vi "Launcher Views.vi"(8 "error in (no error)":errorcluster, 11 "Abstruct View in":refnum<class "Abstruct View.lvclass">) -> (0 "error out":errorcluster, 3 "Abstruct View out":refnum<class "Abstruct View.lvclass">)   [LabVIEW 2020]
uses:
  Abstruct View.lvclass
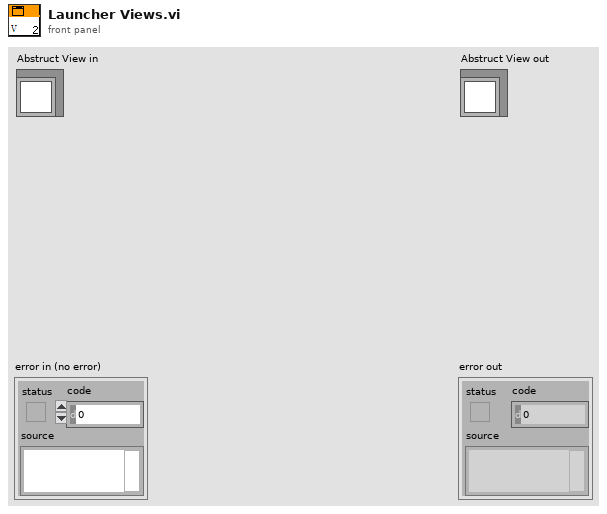
[diagram p1: front panel]
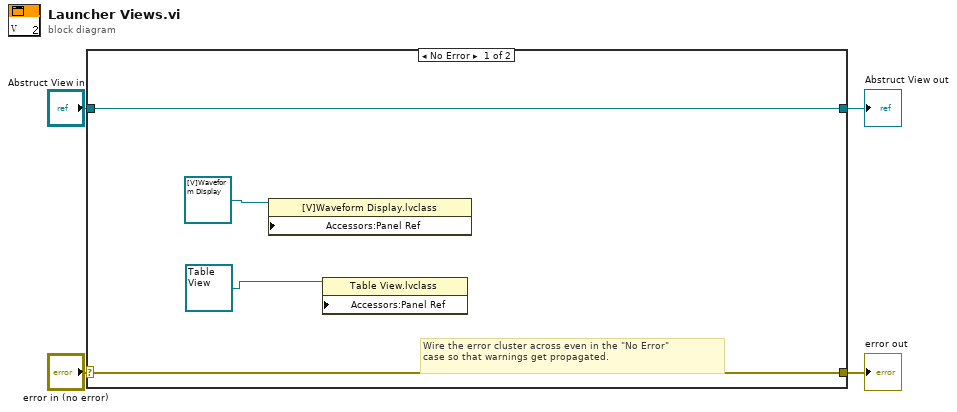
[diagram p0: block diagram]
diagram:
  n1 = case shown="No Error" "error in (no error)" {
    selector: "error in (no error)" -> [w7 w10]
    tunnel: [w7 w10] -> w3
    tunnel: [w8 w9] -> w1
    tunnel: "Abstruct View in" -> [w8 w9]
    frame No Error {
      # "Wire the error cluster across even in the \"No Error\"\ncase so that warnings get propagated."
      n2 = property class="[V]Waveform Display.lvclass" props=["Accessors:Panel Ref"](reference=refnum<class "[V]Waveform Display.lvclass"> refnum ("[V]Waveform Display.lvlib:[V]Waveform Display.lvclass")) -> ()  [unwired: 2 in, 2 out]
      n3 = property class="Table View.lvclass" props=["Accessors:Panel Ref"](reference=refnum<class "Table View.lvclass"> refnum ("[V]Table View.lvlib:Table View.lvclass")) -> ()  [unwired: 2 in, 2 out]
    }
    frame Error {
    }
  }
  "error out" <- w3
  "Abstruct View out" <- w1
